vi "Toggle Torque.vi"(8 "error in (no error)":errorcluster, 9 "Toggle torque (OFF)":bool, 10 "Motor ID (0)":u8, 11 "VISA resource name":refnum<visa-resource-name>) -> (0 "error out":errorcluster, 3 "VISA resource name out":refnum<visa-resource-name>)   [LabVIEW 2016, in "Dynamixel Motor.lvlib"]
doc: "Turns the motor's torque on or off."
uses:
  Dynamixel Motor.lvlib
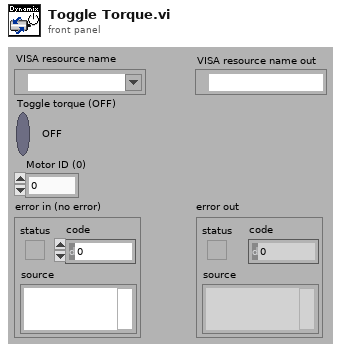
[diagram p1: front panel]
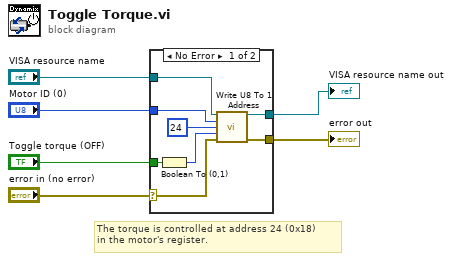
[diagram p0: block diagram]
diagram:
  # "The torque is controlled at address 24 (0x18)\nin the motor's register."
  n1 = case shown="No Error" "error in (no error)" {
    selector: "error in (no error)" -> [w7 w15]
    tunnel: "Toggle torque (OFF)" -> [w12 _]
    tunnel: "VISA resource name" -> [w11 w16]
    tunnel: [w10 w16] -> w4
    tunnel: [w9 w15] -> w3
    tunnel: "Motor ID (0)" -> [w8 _]
    frame No Error {
      n2 = Boolean To (0,1)(Boolean=w12) -> (0, 1=w14:i16)
      n3 = call "Write U8 To 1 Address.vi"("VISA resource name"=w11, "Motor ID (0)"=w8, "Address number (0)"=u8 24, "Parameter (0)"=w14, "error in (no error)"=w7) -> ("VISA resource name out"=w10:refnum<visa-resource-name>, "error out"=w9:errorcluster)  [unwired: 9 in]
    }
    frame Error {
    }
  }
  "VISA resource name out" <- w4
  "error out" <- w3
